vi "Excel Parse Page Info.vi"(8 "[PageLengths]":i32[](array[numeric]), 9 "PageLength":i32=-1, 10 "StartingIndex":i32, 11 "# of Pages":i32) -> (0 "IndexOut":i32, 3 "Page Info":T1(array[cluster]))   [LabVIEW 2019]
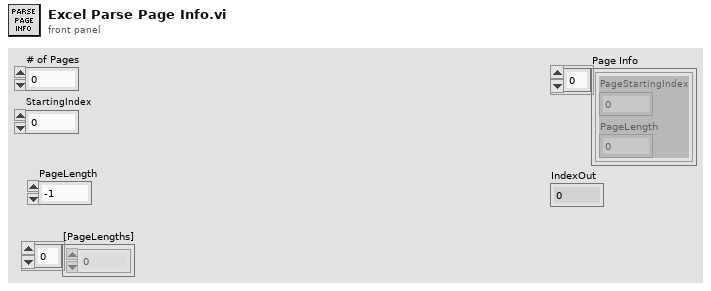
[diagram p1: front panel]
types:
  T1 = cluster{"PageStartingIndex":i32, "PageLength":i32}[]
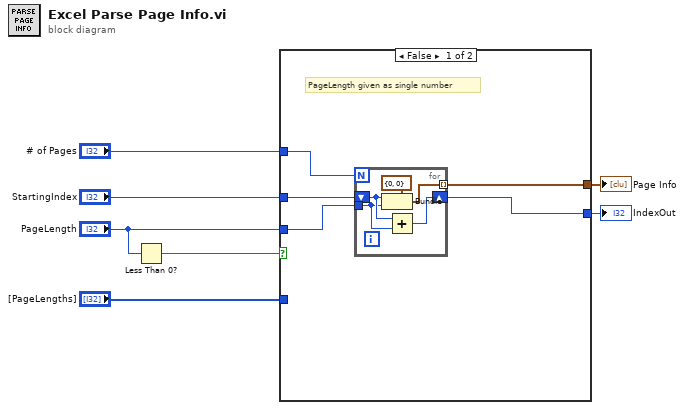
[diagram p0: block diagram]
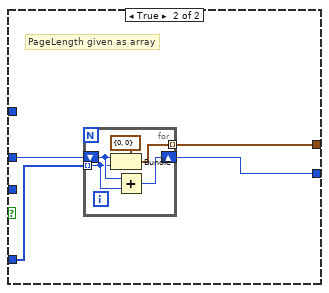
[diagram p2: hidden frame]
diagram:
  n1 = Less Than 0?(x="PageLength") -> (x < 0?=w7:bool)
  n2 = case shown="False" w7 {
    tunnel: "[PageLengths]" -> [_ w21]
    tunnel: "StartingIndex" -> [w12 w20]
    tunnel: "# of Pages" -> [w11 _]
    tunnel: "PageLength" -> [w10 _]
    tunnel: [w9 w19] -> w2
    tunnel: [w8 w18] -> w1
    frame False {
      # "PageLength given as single number"
      n3 = for {
        N: w11 -> [_]
        tunnel: w10 -> [w14]
        shift-right: [w13] -> w8
        shift-left: w12 -> [w15]
        tunnel: [w16] -> w9 mode=indexing
        n4 = Bundle(cluster=cluster{"StartPage":i32, "PageLength":i32} {"StartPage"=0, "PageLength"=0}, "StartPage"=w15, "PageLength"=w14) -> (w16:cluster{"StartPage":i32, "PageLength":i32})
        n5 = Add(x=w15, y=w14) -> (x+y=w13:i32)
      }
    }
    frame True {
      # "PageLength given as array"
      n6 = for {
        tunnel: w21 -> [w23] mode=indexing
        shift-right: [w22] -> w18
        shift-left: w20 -> [w24]
        tunnel: [w25] -> w19 mode=indexing
        n7 = Bundle(cluster=cluster{"StartPage":i32, "PageLength":i32} {"StartPage"=0, "PageLength"=0}, "StartPage"=w24, "PageLength"=w23) -> (w25:cluster{"StartPage":i32, "PageLength":i32})
        n8 = Add(x=w24, y=w23) -> (x+y=w22:i32)
      }
    }
  }
  "Page Info" <- w2
  "IndexOut" <- w1
